vi "Ejercicio_5_Variables_Locales.vi"() -> ()   [LabVIEW 2020]
panel:
  in  "Boolean":bool
  out "Waveform Chart 2":dbl(graph)
  out "Waveform Chart":dbl(graph)
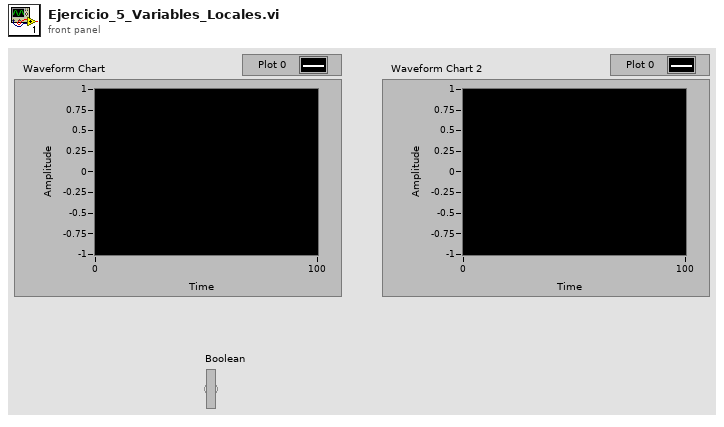
[diagram p1: front panel]
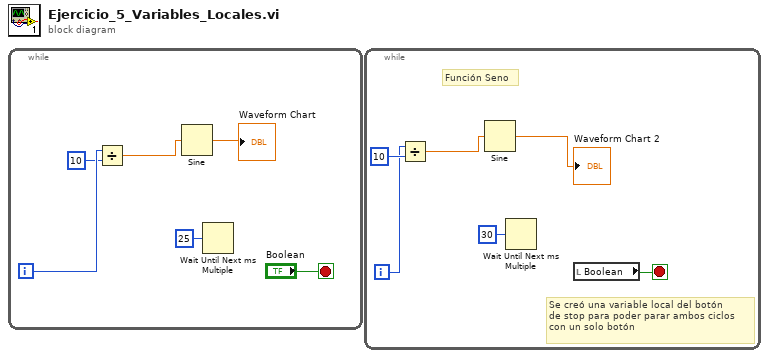
[diagram p0: block diagram]
diagram:
  n1 = while {
    i -> [w5]
    stop <- "Boolean" stop-if-true
    n2 = Divide(x=w5, y=10) -> (x/y=w6:dbl)
    n3 = Sine(x=w6) -> (sin(x)=→"Waveform Chart":dbl)
    n4 = Wait Until Next ms Multiple(millisecond multiple=u32 25) -> ()  [unwired: 1 out]
  }
  n5 = while {
    i -> [w10]
    stop <- w7 stop-if-true
    # "Función Seno"
    # "Se creó una variable local del botón\nde stop para poder parar ambos ciclos \ncon un solo botón"
    n6 = Divide(x=w10, y=10) -> (x/y=w12:dbl)
    n7 = Sine(x=w12) -> (sin(x)=→"Waveform Chart 2":dbl)
    n8 = Wait Until Next ms Multiple(millisecond multiple=u32 30) -> ()  [unwired: 1 out]
    n9 = local read "Boolean"() -> (w7:bool)
  }
